vi "Generate DO DAQ Out Cmd Event.vi"(4 "mode (manual)":T1, 6 "WaitTime (20ms)":u32=20, 8 "error in (no error)":errorcluster, 9 "BoolState":bool, 10 "DO IOName":string, 11 "DAQ":refnum<class "DAQ.lvclass">) -> (0 "error out":errorcluster, 3 "DAQ":refnum<class "DAQ.lvclass">)   [LabVIEW 2017, in "DAQ.lvclass"]
doc: "Developed by Kevin Thompson\nkevin@thompsonengineering.net\n\nCopyright 2018-2020\nThompson Engineering, LLC"
uses:
  DAQ.lvclass
  DataTypes/TD DAQ Output EventSenderMode-enum.ctl
  Process/ProcessSupport/TD DAQ Output Cmd EventData--cluster.ctl
  Process/ProcessSupport/TD DaqOutCmd--enum.ctl
  DAQ.lvclass/DAQ.ctl
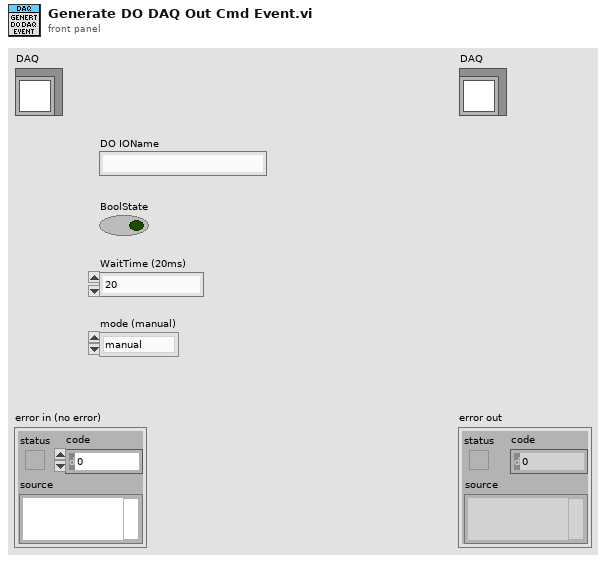
[diagram p1: front panel]
types:
  T1 = typedef "DAQ.lvclass/TD DAQ Output EventSenderMode-enum.ctl" = enum16{"manual", "automation"}
  T2 = typedef "DAQ.lvclass/TD DaqOutCmd--enum.ctl" = enum16{"Set DO", "Set AO", "Toggle DO"}
  T3 = typedef "DAQ.lvclass/TD DAQ Output Cmd EventData--cluster.ctl" = cluster{"TimeStamp":dbl, "DaqOutCmd":T2, "IOName":string, "BoolState":bool, "AnalogVal":dbl, "WaitTime (ms)":u32, "mode":T1, "vData":variant}
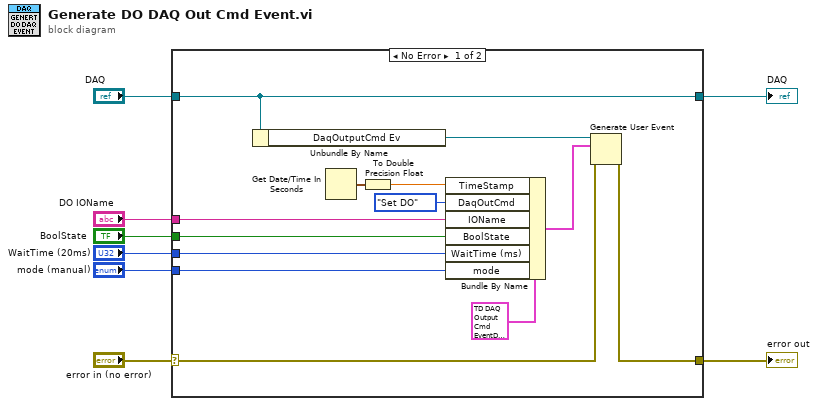
[diagram p0: block diagram]
diagram:
  n1 = case shown="No Error" "error in (no error)" {
    selector: "error in (no error)" -> [w13 w23]
    tunnel: [w12 w23] -> w7
    tunnel: [w21 w22] -> w5
    tunnel: "DAQ" -> [w21 w22]
    tunnel: "DO IOName" -> [w9 _]
    tunnel: "WaitTime (20ms)" -> [w14 _]
    tunnel: "BoolState" -> [w11 _]
    tunnel: "mode (manual)" -> [w10 _]
    frame No Error {
      n2 = Unbundle By Name(w21) -> ("DaqOutputCmd Ev"=w20:refnum<user-event>)
      n3 = Get Date/Time In Seconds() -> (seconds since 1Jan1904=w17:timestamp)
      n4 = To Double Precision Float(number=w17) -> (double precision float=w16:dbl)
      n5 = Bundle By Name(cluster=T3 {"TimeStamp"=0.0, "DaqOutCmd"=enum."Set DO", "IOName"="", "BoolState"=FALSE, "AnalogVal"=0.0, "WaitTime (ms)"=0, "mode"=enum."manual", "vData"=variant} ("DaqOutputCmd"), "TimeStamp"=w16, "DaqOutCmd"=TD_DaqOutCmd--enum."Set DO", "IOName"=w9, "BoolState"=w11, "WaitTime (ms)"=w14, "mode"=w10) -> (w18:T3)
      n6 = Generate User Event(user event=w20, event data cluster=w18, error in=w13) -> (error out=w12:errorcluster)  [unwired: 1 in, 1 out]
    }
    frame Error {
    }
  }
  "error out" <- w7
  "DAQ" <- w5
